vi "AppendImageToReport_Mutation.vi"(0 "Diagram":refnum<vi>, 5 "ObjRef":refnum<vi>, 6 "Kind":string="SubVI", 7 "Information":string="<Not A Path>") -> (3 "Replace?":bool)   [LabVIEW 2020]
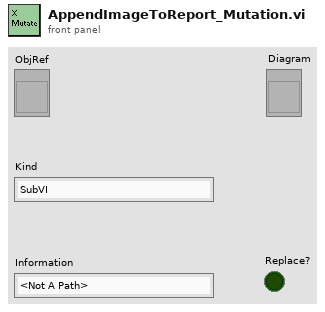
[diagram p1: front panel]
types:
  T1 = typedef "LVPositionTypeDef.ctl" = cluster{"Left":i32, "Top":i32}
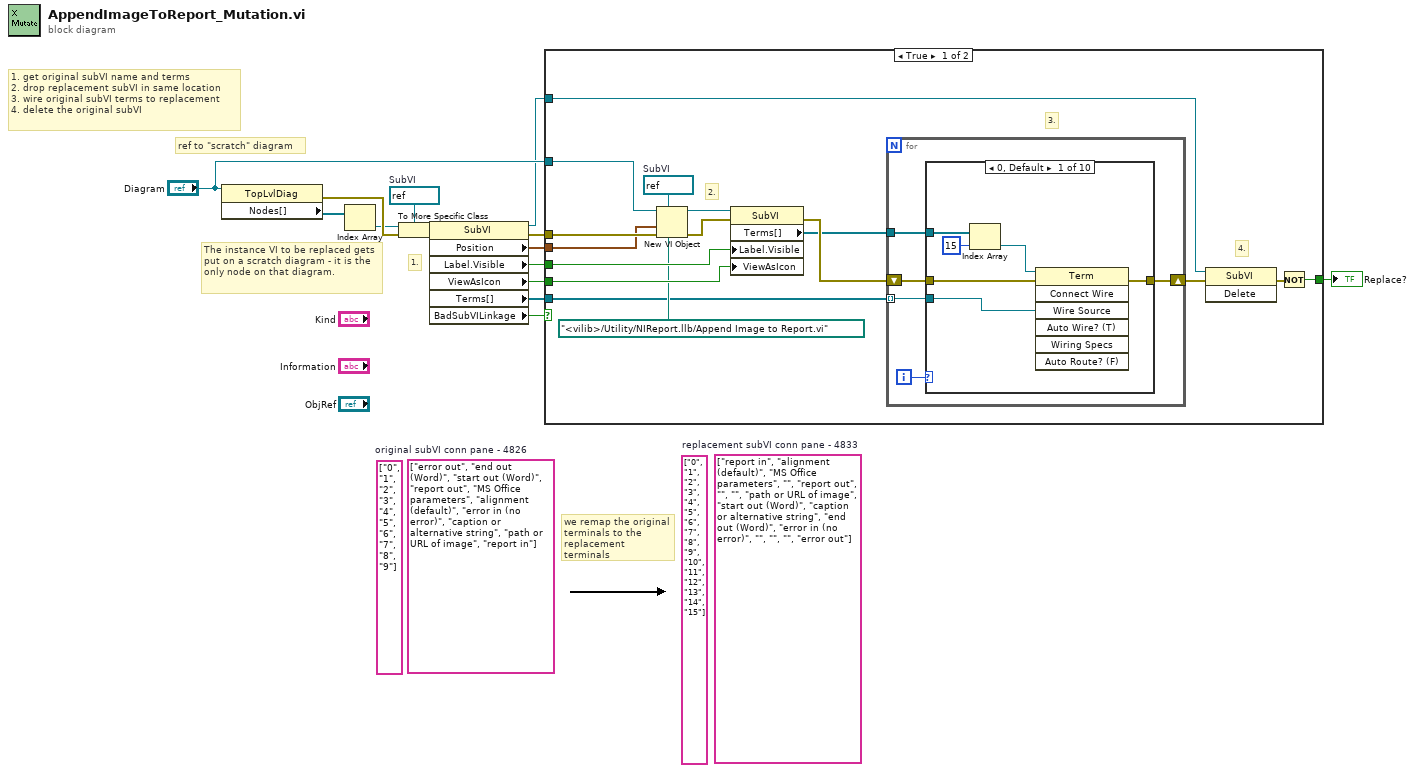
[diagram p0: block diagram]
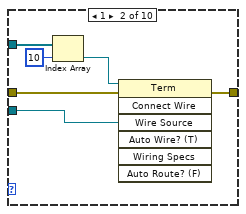
[diagram p2: hidden frame]
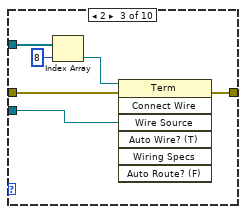
[diagram p3: hidden frame]
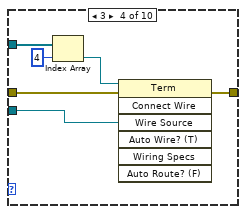
[diagram p4: hidden frame]
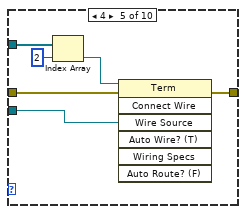
[diagram p5: hidden frame]
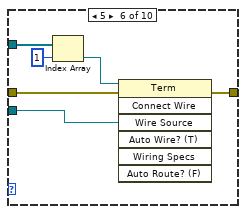
[diagram p6: hidden frame]
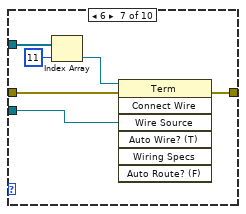
[diagram p7: hidden frame]
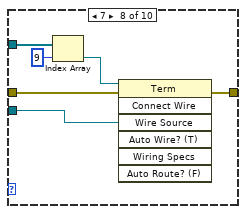
[diagram p8: hidden frame]
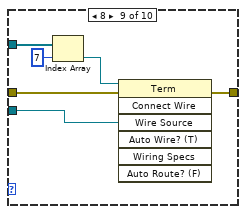
[diagram p9: hidden frame]
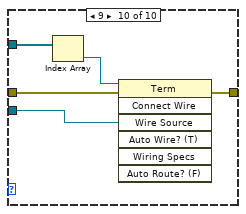
[diagram p10: hidden frame]
diagram:
  (unwired) string[] ["0", "1", "2", "3", "4", "5", "6", "7", "8", "9", "10", "11", "12", "13", "14", "15"]
  (unwired) string[] ["0", "1", "2", "3", "4", "5", "6", "7", "8", "9"]
  (unwired) string[] ["report in", "alignment (default)", "MS Office parameters", "", "report out", "", "", "path or URL of image", "start out (Word)", "caption or alternative string", "end out (Word)", "error in (no error)", "", "", "", "error out"]  # replacement subVI conn pane - 4833
  (unwired) string[] ["error out", "end out (Word)", "start out (Word)", "report out", "MS Office parameters", "alignment (default)", "error in (no error)", "caption or alternative string", "path or URL of image", "report in"]  # original subVI conn pane - 4826
  w12 = refnum<vi> refnum  # SubVI
  # "1."
  # "we remap the original terminals to the replacement terminals"
  # "The instance VI to be replaced gets put on a scratch diagram - it is the only node on that diagram."
  # "1. get original subVI name and terms\n2. drop replacement subVI in same location\n3. wire original subVI terms to replacement\n4. delete the original subVI"
  # "ref to \"scratch\" diagram"
  n1 = property class="TopLvlDiag"(reference="Diagram") -> (error out=w14:errorcluster, "Nodes[]"=w10:refnum<vi>[])  [unwired: 1 in, 1 out]
  n2 = Index Array(array=w10) -> (element=w9:refnum<vi>)  [unwired: 1 in]
  n3 = To More Specific Class(target class=w12, reference=w9, error in=w14) -> (specific class reference=w11:refnum<vi>, error out=w15:errorcluster)
  n4 = property class="SubVI"(reference=w11, error in=w15) -> (reference out=w4:refnum<vi>, error out=w13:errorcluster, "Position"=w5:T1, "Label.Visible"=w8:bool, "ViewAsIcon"=w7:bool, "Terms[]"=w2:refnum<vi>[], "BadSubVILinkage"=w1:bool)
  n5 = case shown="True" w1 {
    tunnel: w8 -> [w24 _]
    tunnel: w7 -> [w23 _]
    tunnel: "Diagram" -> [w22 _]
    tunnel: w5 -> [w21 _]
    tunnel: w4 -> [w20 _]
    tunnel: [w19 _] -> w3
    tunnel: w13 -> [w30 _]
    tunnel: w2 -> [w16 _]
    frame True {
      w26 = refnum<vi> refnum  # SubVI
      # "4."
      # "3."
      # "2."
      n6 = New VI Object(vi object class=w26, owner refnum=w22, position/next to=w21, 6:path "<vilib>/Utility/NIReport.llb/Append Image to Report.vi", 8:w30) -> (object refnum=w25:refnum<vi>, 0:w29:errorcluster)  [unwired: 3 in]
      n7 = property class="SubVI"(reference=w25, error in=w29, "Label.Visible"=w24, "ViewAsIcon"=w23) -> (error out=w28:errorcluster, "Terms[]"=w17:refnum<vi>[])  [unwired: 1 out]
      n8 = for {
        tunnel: w16 -> [w33] mode=indexing
        tunnel: w17 -> [w32]
        shift-right: [w35] -> w31
        shift-left: w28 -> [w36]
        i -> [w34]
        n9 = case shown="0, Default" w34 {
          tunnel: w33 -> [w40 w46 w52 w58 w64 w70 w76 w82 w88 w93]
          tunnel: w32 -> [w39 w45 w51 w57 w63 w69 w75 w81 w87 w92]
          tunnel: w36 -> [w42 w48 w54 w60 w66 w72 w78 w84 w90 w95]
          tunnel: [w41 w47 w53 w59 w65 w71 w77 w83 w89 w94] -> w35
          frame 0, Default {
            n10 = Index Array(array=w39, index=15) -> (element=w37:refnum<vi>)
            n11 = invoke class="Term" method="Connect Wire"(reference=w37, error in=w42, "Wire Source"=w40) -> (error out=w41:errorcluster)  [unwired: 4 in, 6 out]
          }
          frame 1 {
            n12 = Index Array(array=w45, index=10) -> (element=w43:refnum<vi>)
            n13 = invoke class="Term" method="Connect Wire"(reference=w43, error in=w48, "Wire Source"=w46) -> (error out=w47:errorcluster)  [unwired: 4 in, 6 out]
          }
          frame 2 {
            n14 = Index Array(array=w51, index=8) -> (element=w49:refnum<vi>)
            n15 = invoke class="Term" method="Connect Wire"(reference=w49, error in=w54, "Wire Source"=w52) -> (error out=w53:errorcluster)  [unwired: 4 in, 6 out]
          }
          frame 3 {
            n16 = Index Array(array=w57, index=4) -> (element=w55:refnum<vi>)
            n17 = invoke class="Term" method="Connect Wire"(reference=w55, error in=w60, "Wire Source"=w58) -> (error out=w59:errorcluster)  [unwired: 4 in, 6 out]
          }
          frame 4 {
            n18 = Index Array(array=w63, index=2) -> (element=w61:refnum<vi>)
            n19 = invoke class="Term" method="Connect Wire"(reference=w61, error in=w66, "Wire Source"=w64) -> (error out=w65:errorcluster)  [unwired: 4 in, 6 out]
          }
          frame 5 {
            n20 = Index Array(array=w69, index=1) -> (element=w67:refnum<vi>)
            n21 = invoke class="Term" method="Connect Wire"(reference=w67, error in=w72, "Wire Source"=w70) -> (error out=w71:errorcluster)  [unwired: 4 in, 6 out]
          }
          frame 6 {
            n22 = Index Array(array=w75, index=11) -> (element=w73:refnum<vi>)
            n23 = invoke class="Term" method="Connect Wire"(reference=w73, error in=w78, "Wire Source"=w76) -> (error out=w77:errorcluster)  [unwired: 4 in, 6 out]
          }
          frame 7 {
            n24 = Index Array(array=w81, index=9) -> (element=w79:refnum<vi>)
            n25 = invoke class="Term" method="Connect Wire"(reference=w79, error in=w84, "Wire Source"=w82) -> (error out=w83:errorcluster)  [unwired: 4 in, 6 out]
          }
          frame 8 {
            n26 = Index Array(array=w87, index=7) -> (element=w85:refnum<vi>)
            n27 = invoke class="Term" method="Connect Wire"(reference=w85, error in=w90, "Wire Source"=w88) -> (error out=w89:errorcluster)  [unwired: 4 in, 6 out]
          }
          frame 9 {
            n28 = Index Array(array=w92) -> (element=w91:refnum<vi>)  [unwired: 1 in]
            n29 = invoke class="Term" method="Connect Wire"(reference=w91, error in=w95, "Wire Source"=w93) -> (error out=w94:errorcluster)  [unwired: 4 in, 6 out]
          }
        }
      }
      n30 = invoke class="SubVI" method="Delete"(reference=w20, error in=w31) -> (error out=w27:errorcluster)  [unwired: 1 in, 2 out]
      n31 = Not(x=w27) -> (.not. x?=w19:bool)
    }
    frame False {
    }
  }
  "Replace?" <- w3
